vi "updateMDF.vi"(6 "Behaviors":T1(ring), 7 "MDF":T2(array[cluster]), 8 "MDF Index to Change":i32, 9 "Speed":i32, 10 "Y new wp":i32, 11 "X new wp":i32) -> (5 "New MDF":T2(array[cluster]))   [LabVIEW 2014]
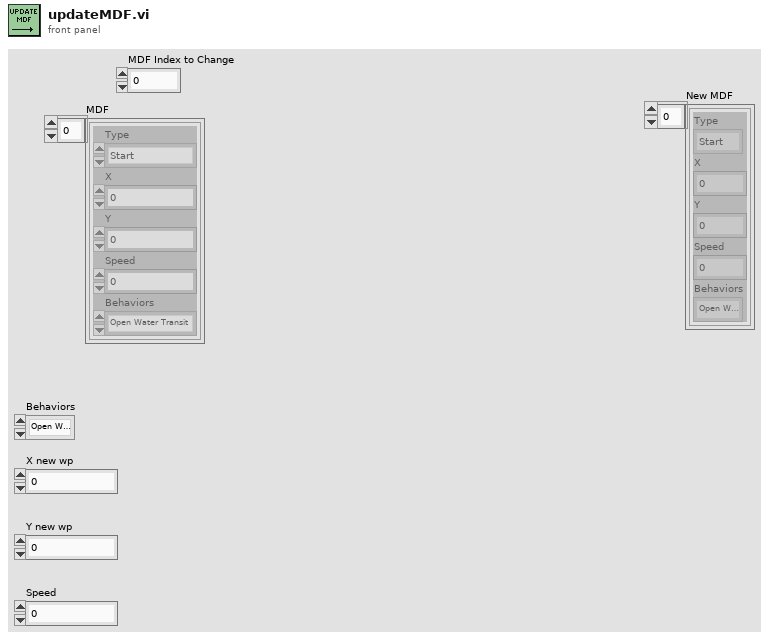
[diagram p1: front panel]
types:
  T1 = enum16{"Open Water Transit", "P-Wall Follow", "S-Wall Follow", "Get Unstuck"}
  T2 = cluster{"Type":enum16{"Start", "Buoy Circling", "Waypoint", "End"}, "X":i32, "Y":i32, "Speed":i32, "Behaviors":enum16{"Open Water Transit", "P-Wall Follow", "S-Wall Follow", "Get Unstuck"}}[]
  T3 = enum16{"Start", "Buoy Circling", "Waypoint", "End"}
  T4 = cluster{"Type":enum16{"Start", "Buoy Circling", "Waypoint", "End"}, "X new wp":i32, "Y new wp":i32, "Speed":i32, "Behaviors":enum16{"Open Water Transit", "P-Wall Follow", "S-Wall Follow", "Get Unstuck"}}
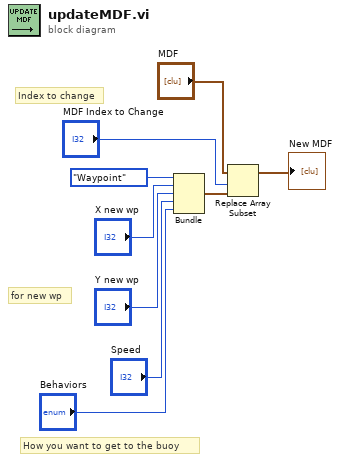
[diagram p0: block diagram]
diagram:
  # "How you want to get to the buoy"
  # "for new wp"
  # "Index to change"
  n1 = Bundle("Type"=T3."Waypoint", "X new wp"="X new wp", "Y new wp"="Y new wp", "Speed"="Speed", "Behaviors"="Behaviors") -> (w2:T4)  [unwired: 1 in]
  n2 = Replace Array Subset(array="MDF", new element=w2, index="MDF Index to Change") -> (→"New MDF":T2)
